vi "Burner.vi"(11 "Port":string) -> ()   [LabVIEW 2020]
panel:
  out "length":i32
  out "OUTPUT CONSOLE":string
  out "ERROR":string
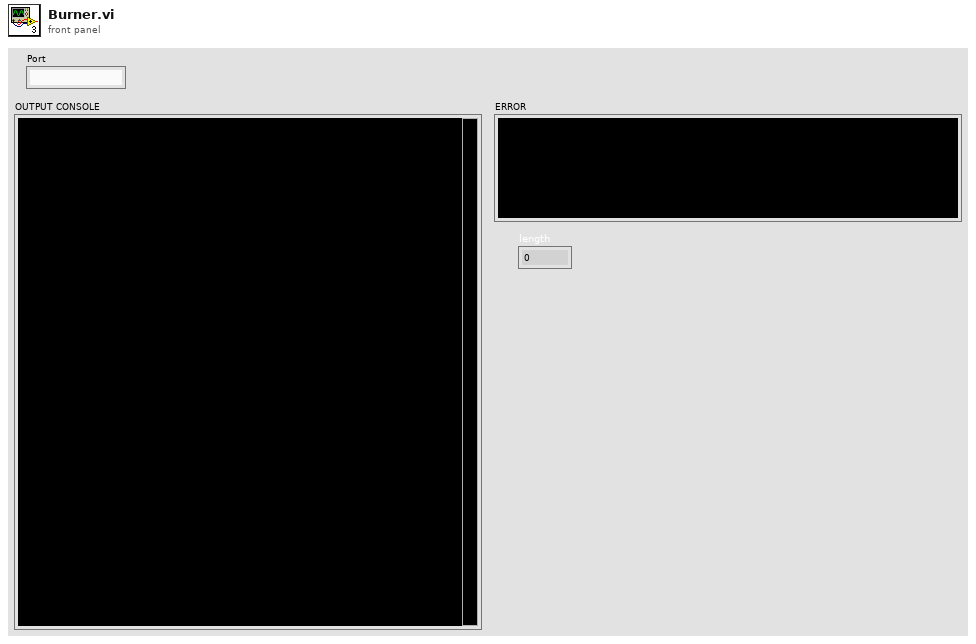
[diagram p1: front panel]
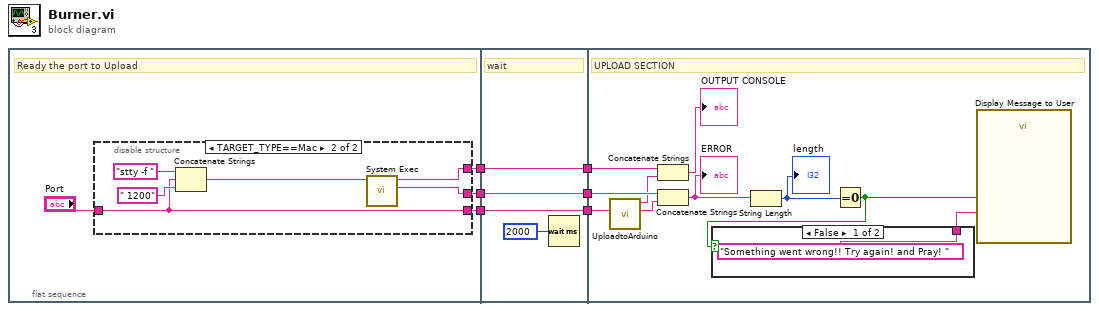
[diagram p0: block diagram]
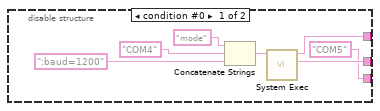
[diagram p2: hidden frame]
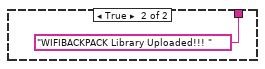
[diagram p3: hidden frame]
diagram:
  n1 = flat-sequence {
    tunnel: [w8] -> w6
    tunnel: [w9] -> w3
    tunnel: [w10] -> w2
    tunnel: w6 -> [w26]
    tunnel: [w26] -> w5
    tunnel: [w25] -> w4
    tunnel: w3 -> [w25]
    tunnel: w2 -> [w24]
    tunnel: [w24] -> w1
    tunnel: w5 -> [w32]
    tunnel: w4 -> [w37]
    tunnel: w1 -> [w35]
    frame #0 {
      # "Ready the port to Upload"
      n2 = disable-structure shown="TARGET_TYPE==Mac" {
        disable-tunnel: [w13 w20] -> w10
        disable-tunnel: [w12 w19] -> w9
        disable-tunnel: ["COM5" ("string") w18] -> w8
        disable-tunnel: "Port" -> [_ w18]
        frame condition #0 {
          n3 = Concatenate Strings("mode" ("string"), "COM4" ("string"), ":baud=1200" ("string")) -> (w17:string)
          n4 = call <vilib>:"System Exec.vi"("command line"=w17) -> ("standard error"=w12:string, "standard output"=w13:string)  [unwired: 7 in, 2 out]
        }
        frame condition #1 (active) {
          n5 = Concatenate Strings("stty -f " ("string"), w18, " 1200" ("string")) -> (w23:string)
          n6 = call <vilib>:"System Exec.vi"("command line"=w23) -> ("standard error"=w19:string, "standard output"=w20:string)  [unwired: 7 in, 2 out]
        }
      }
    }
    frame #1 {
      # "wait"
      n7 = Wait (ms)(milliseconds to wait=u32 2000) -> ()  [unwired: 1 out]
    }
    frame #2 {
      # "UPLOAD SECTION"
      n8 = call "UploadtoArduino.vi"("serial port"=w32) -> ("standard error"=w36:string, "standard output"=w34:string)  [unwired: 9 in]
      n9 = Concatenate Strings(w35, w34) -> (→"OUTPUT CONSOLE":string)
      n10 = Concatenate Strings(w37, w36) -> (w31:string)
      "ERROR" <- w31
      n11 = String Length(string=w31) -> (length=w30:i32)
      "length" <- w30
      n12 = Equal To 0?(x=w30) -> (x = 0?=w28:bool)
      n13 = case shown="False" w28 {
        tunnel: ["Something went wrong!! Try again! and Pray! " "WIFIBACKPACK Library Uploaded!!! "] -> w29
        frame False {
        }
        frame True {
        }
      }
      n14 = call "Display Message to User"("Enable"=w28, "Message"=w29) -> ()  [unwired: 8 in, 2 out]
    }
  }
